vi "Test Reentrant VI Calls are Indistinguishable.vi"(8 "error in (no error)":errorcluster, 11 "Test Case In":refnum<class "One Expectation Test.lvclass">) -> (0 "error out":errorcluster, 3 "Test Case Out":refnum<class "One Expectation Test.lvclass">)   [LabVIEW 2020, in "One Expectation Test.lvclass"]
uses:
  One Expectation Test.lvclass
  C:/Program Files (x86)/National Instruments/LabVIEW 2020/vi.lib/Astemes/LUnit/Test Case.lvclass
  Indentical Inputs Comparator/Identical Inputs Comparator.lvclass
  C:/git/astemes-lmock/sandbox/Comparator/Comparator.lvclass
  Test Interface Mock/Test Interface Mock.lvclass
  C:/git/astemes-lmock/sandbox/Mock/Mock.lvclass
  One Of/One.lvclass
  Expectation Test/Expectation Test.lvclass
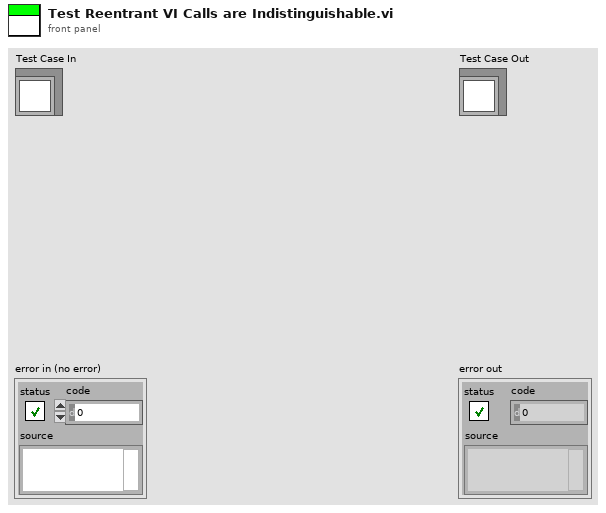
[diagram p1: front panel]
types:
  T1 = enum16{"", "Passed", "Failed", "Error", "Skipped", "Setup Error", "Broken", "Teardown Error"}
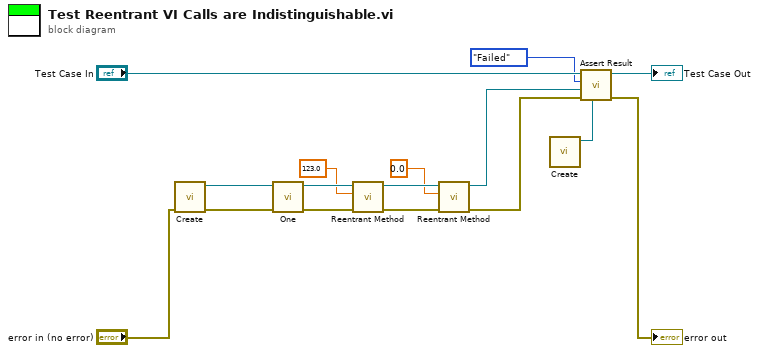
[diagram p0: block diagram]
diagram:
  n1 = call "Create.vi"("error in (no error)"="error in (no error)") -> ("error out"=w15:errorcluster, "Test Interface Mock Out"=w16:refnum<class "Test Interface Mock.lvclass">)  [unwired: 9 in]
  n2 = call "One.vi"("error in (no error)"=w15, "Mock in"=w16) -> ("error out"=w13:errorcluster, "Mock out"=w14:refnum<class "Test Interface Mock.lvclass">)  [unwired: 8 in]
  n3 = call-dynamic "Reentrant Method.vi"("error in (no error)"=w13, "Numeric"=123.0, "Test Interface Mock in"=w14) -> ("error out"=w12:errorcluster, "Test Interface Mock out"=w6:refnum<class "Test Interface Mock.lvclass">)  [unwired: 7 in]
  n4 = call-dynamic "Reentrant Method.vi"("error in (no error)"=w12, "Numeric"=0.0, "Test Interface Mock in"=w6) -> ("error out"=w7:errorcluster, "Test Interface Mock out"=w4:refnum<class "Test Interface Mock.lvclass">)  [unwired: 7 in]
  n5 = call "Create.vi"() -> ("Identical Inputs Comparator"=w1:refnum<class "Identical Inputs Comparator.lvclass">)  [unwired: 10 in, 1 out]
  n6 = call "Assert Result.vi"("Comparator"=w1, "error in (no error)"=w7, "Mock"=w4, "Status"=T1."Failed", "LUnit Test Case In"="Test Case In") -> ("error out"=→"error out":errorcluster, "LUnit Test Case Out"=→"Test Case Out":refnum<class "One Expectation Test.lvclass">)  [unwired: 5 in]
